vi "Axis_Offset.vi"(3 "Position In":sgl[](array[numeric])=[0.0, 0.0, 0.0] format="%#.2f", 4 "Axis":T1, 5 "Roll-Pitch-Yaw":sgl[](array[numeric]) caption="Model       Roll         Pitch        Yaw (deg)" format="%#.2f", 6 "Traverse Name":string) -> (0 "Correct array":bool, 1 "Offset":sgl, 2 "Offset Array":sgl[](array[numeric]))   [LabVIEW 2022 SP3]
uses:
  Route mapping/Axis.ctl
  Globals/Constants_global.vi
  Globals/Trav_pos_global.vi
  Globals/Meas_global.vi
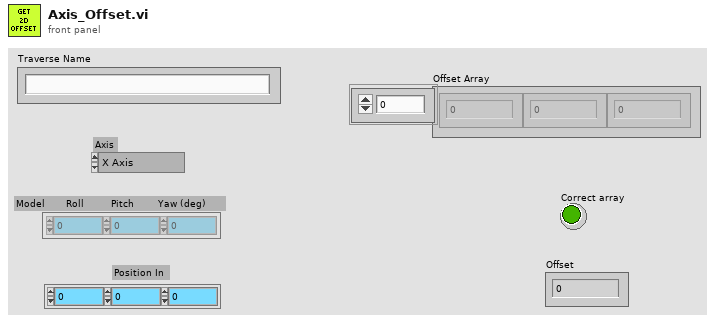
[diagram p1: front panel]
types:
  T1 = typedef "Axis.ctl" = enum16{"X Axis", "X Axis -ve", "Y Axis", "Y Axis -ve", "Z Axis", "Z Axis -ve"}
  T2 = enum16{"To Traverse Coordinates", "To User Coordinates"}
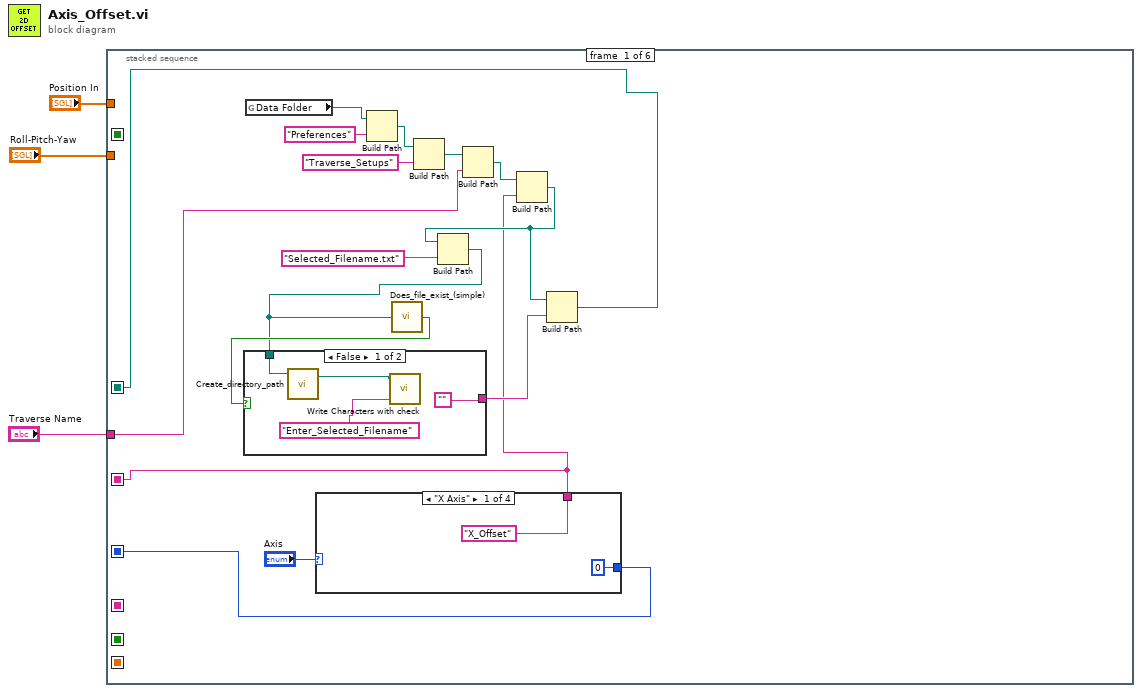
[diagram p0: block diagram]
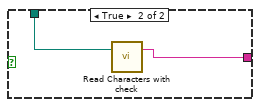
[diagram p2: hidden frame]
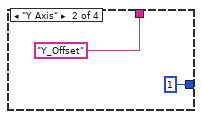
[diagram p3: hidden frame]
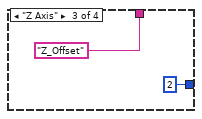
[diagram p4: hidden frame]
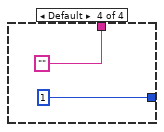
[diagram p5: hidden frame]
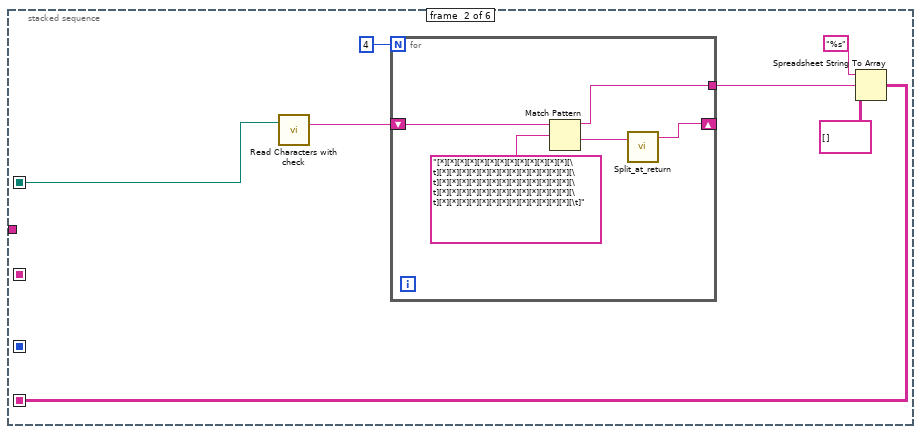
[diagram p6: hidden frame]
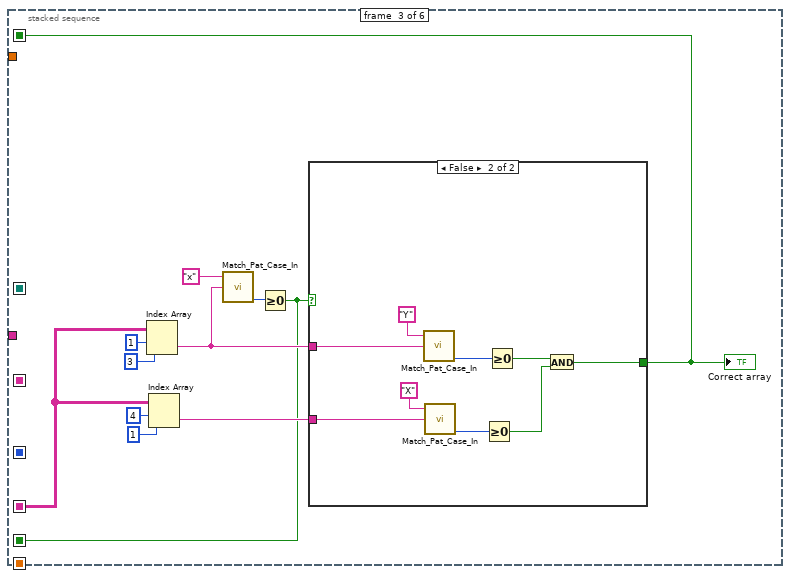
[diagram p7: hidden frame]
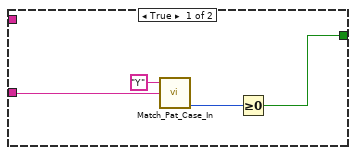
[diagram p8: hidden frame]
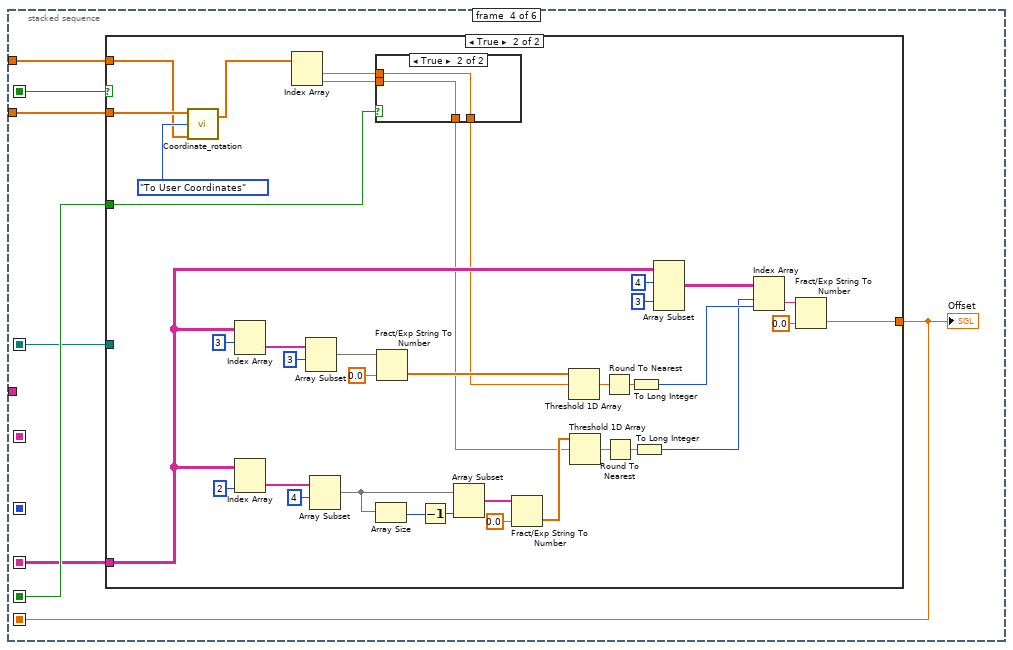
[diagram p9: hidden frame]
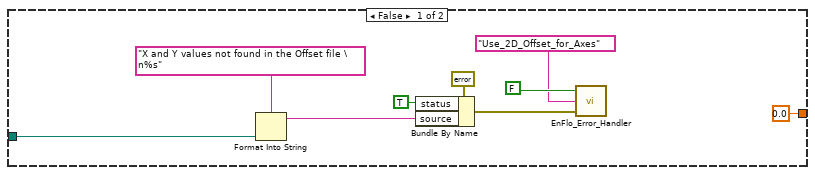
[diagram p10: hidden frame]
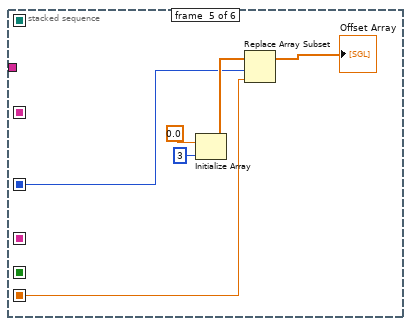
[diagram p12: hidden frame]
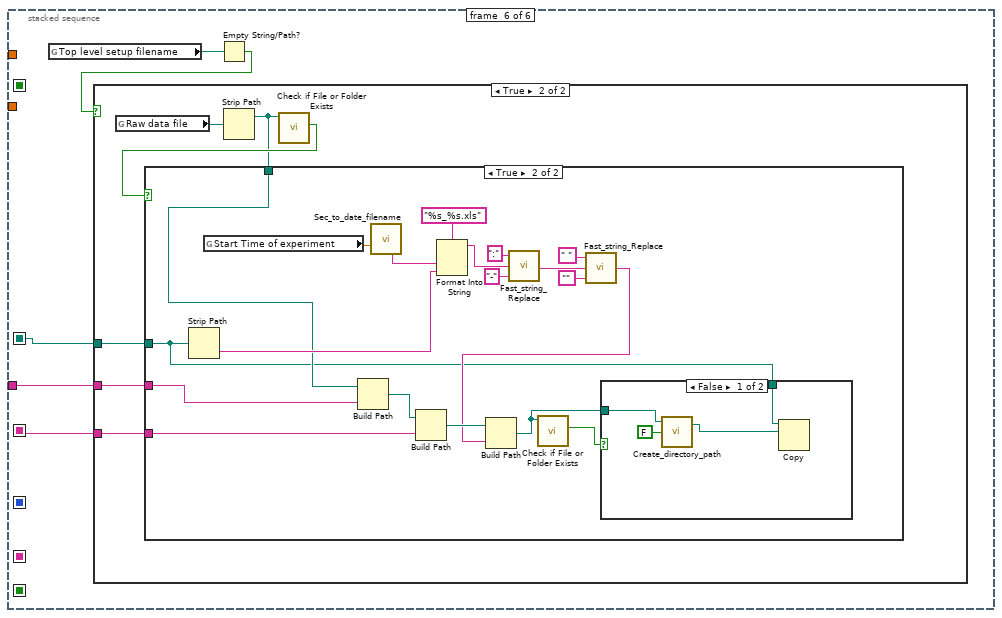
[diagram p13: hidden frame]
diagram:
  n1 = stacked-sequence {
    seq-local: [_ w36 _ _ _ _] -> [_ _ w51 w71 _ _]
    seq-local: [_ _ w47 _ _ _] -> [_ _ _ w76 _ _]
    seq-local: [_ _ _ w73 _ _] -> [_ _ _ _ w127 _]
    seq-local: [_ _ w46 _ _ _] -> [_ _ _ w74 _ _]
    seq-local: [w7 _ _ _ _ _] -> [_ w35 _ w72 _ w135]
    seq-local: [w6 _ _ _ _ _] -> [_ _ _ _ w129 _]
    seq-local: [w4 _ _ _ _ _] -> [_ _ _ _ _ w133]
    tunnel: "Position In" -> [_ _ _ w75 _ _]
    tunnel: "Roll-Pitch-Yaw" -> [_ _ _ w70 _ _]
    tunnel: "Traverse Name" -> [w5 _ _ _ _ w134]
    frame #0 {
      n2 = global read "Constants_global.vi" "Data Folder"() -> (w9:path)
      n3 = case shown="\"X Axis\"" "Axis" {
        tunnel: ["X_Offset" ("name or relative path") "Y_Offset" ("name or relative path") "Z_Offset" ("name or relative path") "" ("name or relative path")] -> w4
        tunnel: [0 ("index") 1 ("index") 2 ("index") 1 ("index")] -> w6
        frame "X Axis" {
        }
        frame "Y Axis" {
        }
        frame "Z Axis" {
        }
        frame Default {
        }
      }
      n4 = Build Path(base path=w9, name or relative path="Preferences") -> (appended path=w11:path)
      n5 = Build Path(base path=w11, name or relative path="Traverse_Setups") -> (appended path=w12:path)
      n6 = Build Path(base path=w12, name or relative path=w5) -> (appended path=w15:path)
      n7 = Build Path(base path=w15, name or relative path=w4) -> (appended path=w16:path)
      n8 = Build Path(base path=w16, name or relative path="Selected_Filename.txt" ("Substring")) -> (appended path=w17:path)
      n9 = call "Does_file_exist_(simple).vi"("Pathname"=w17) -> ("exists?"=w18:bool)
      n10 = case shown="False" w18 {
        tunnel: w17 -> [w23 w25]
        tunnel: ["" w24] -> w19
        frame False {
          n11 = call "Create_directory_path.vi"("Path name"=w23) -> ("Path name Out"=w21:path)  [unwired: 2 in, 1 out]
          n12 = call "Write Characters with check.vi"("String to Write"="Enter_Selected_Filename" ("Substring"), "file (use dialog)"=w21) -> ()  [unwired: 2 in, 1 out]
        }
        frame True {
          n13 = call "Read Characters with check.vi"("file (use dialog)"=w25) -> ("Read String"=w24:string)  [unwired: 1 in, 1 out]
        }
      }
      n14 = Build Path(base path=w16, name or relative path=w19) -> (appended path=w7:path)
    }
    frame #1 {
      n15 = call "Read Characters with check.vi"("file (use dialog)"=w35) -> ("Read String"=w34:string)  [unwired: 1 in, 1 out]
      n16 = for {
        N: 4 -> [_]
        shift-right: [w42] -> _
        shift-left: w34 -> [w43]
        tunnel: [w41] -> w38
        n17 = Match Pattern(string=w43, regular expression="[*][*][*][*][*][*][*][*][*][*][*][*][*][\t][*][*][*][*][*][*][*][*][*][*][*][*][*][\t][*][*][*][*][*][*][*][*][*][*][*][*][*][\t][*][*][*][*][*][*][*][*][*][*][*][*][*][\t][*][*][*][*][*][*][*][*][*][*][*][*][*][\t]" ("String")) -> (before substring=w41:string, after substring=w44:string)  [unwired: 3 out]
        n18 = call "Split_at_return.vi"("String"=w44) -> ("after substring"=w42:string)  [unwired: 1 in, 3 out]
      }
      n19 = Spreadsheet String To Array(format string="%s", spreadsheet string=w38, array type (2D Dbl)=string[][] []) -> (array=w36:string[][])  [unwired: 1 in]
    }
    frame #2 {
      n20 = Index Array(array=w51, index (row)=1, index (col)=3) -> (element=w49:string)
      n21 = Index Array(array=w51, index (row)=4, index (col)=1) -> (element=w50:string)
      n22 = call "Match_Pat_Case_In.vi"("String to match"="x", "String"=w49) -> ("offset past match"=w48:i32)  [unwired: 1 in, 3 out]
      n23 = Greater Or Equal To 0?(x=w48) -> (x >= 0?=w47:bool)
      n24 = case shown="False" w47 {
        tunnel: w50 -> [w59 w68]
        tunnel: w49 -> [_ w66]
        tunnel: [w57 w61] -> w46
        frame True {
          n25 = call "Match_Pat_Case_In.vi"("String to match"="Y", "String"=w59) -> ("offset past match"=w58:i32)  [unwired: 1 in, 3 out]
          n26 = Greater Or Equal To 0?(x=w58) -> (x >= 0?=w57:bool)
        }
        frame False {
          n27 = call "Match_Pat_Case_In.vi"("String to match"="Y", "String"=w66) -> ("offset past match"=w65:i32)  [unwired: 1 in, 3 out]
          n28 = call "Match_Pat_Case_In.vi"("String to match"="X", "String"=w68) -> ("offset past match"=w64:i32)  [unwired: 1 in, 3 out]
          n29 = Greater Or Equal To 0?(x=w64) -> (x >= 0?=w63:bool)
          n30 = Greater Or Equal To 0?(x=w65) -> (x >= 0?=w62:bool)
          n31 = And(x=w62, y=w63) -> (x .and. y?=w61:bool)
        }
      }
      "Correct array" <- w46
    }
    frame #3 {
      n32 = case shown="True" w74 {
        tunnel: w71 -> [_ w108]
        tunnel: w76 -> [_ w107]
        tunnel: [sgl 0.0 w102] -> w73
        tunnel: w75 -> [_ w87]
        tunnel: w72 -> [w79 _]
        tunnel: w70 -> [_ w88]
        frame False {
          n33 = Format Into String(format string="X and Y values not found in the Offset file \n%s", w79) -> (resulting string=w77:string)  [unwired: 2 in, 1 out]
          n34 = Bundle By Name(cluster=errorcluster {"status"=FALSE, "code"=0, "source"=""} ("error in (no error)"), "status"=TRUE, "source"=w77) -> (w82:errorcluster)
          n35 = call "EnFlo_Error_Handler.vi"("error in (no error)"=w82, "Error Type"="Use_2D_Offset_for_Axes", "Dialog Box (F)"=FALSE ("Dialog Box (T)")) -> ()  [unwired: 1 in, 2 out]
        }
        frame True {
          n36 = call "Coordinate_rotation.vi"("Roll-Pitch-Yaw"=w88, "Input Position"=w87, "Mode"=T2."To User Coordinates") -> ("Output Position"=w86:sgl[])  [unwired: 2 in, 1 out]
          n37 = Index Array(array=w108, index (row)=3) -> (element=w121:string[])  [unwired: 1 in]
          n38 = Index Array(array=w108, index (col)=2 ("index (row)")) -> (element=w117:string[])  [unwired: 1 in]
          n39 = Index Array(array=w86) -> (element #1=w104:sgl, element #2=w103:sgl)  [unwired: 2 in]
          n40 = Array Subset(array=w121, index=3) -> (w114:string[])  [unwired: 1 in]
          n41 = Array Subset(array=w117, index=4) -> (w94:string[])  [unwired: 1 in]
          n42 = case shown="True" w107 {
            tunnel: w104 -> [w124 w126]
            tunnel: [w123 w126] -> w106
            tunnel: [w124 w125] -> w105
            tunnel: w103 -> [w123 w125]
            frame False {
            }
            frame True {
            }
          }
          n43 = Array Size(array=w94) -> (size(s)=w96:i32)
          n44 = Fract/Exp String To Number(string=w114, default (0 dbl)=sgl 0.0 ("default (0 DBL)")) -> (number=w113:sgl[])  [unwired: 2 in, 1 out]
          n45 = Decrement(x=w96) -> (x-1=w95:i32)
          n46 = Array Subset(array=w94, length=w95) -> (w93:string[])  [unwired: 1 in]
          n47 = Fract/Exp String To Number(string=w93, default (0 dbl)=sgl 0.0 ("default (0 DBL)")) -> (number=w110:sgl[])  [unwired: 2 in, 1 out]
          n48 = Threshold 1D Array(2:w106, 3:w113) -> (0:w112:sgl)  [unwired: 1 in]
          n49 = Threshold 1D Array(2:w105, 3:w110) -> (0:w111:sgl)  [unwired: 1 in]
          n50 = Round To Nearest(number=w112) -> (nearest integer value=w101:sgl)
          n51 = Round To Nearest(number=w111) -> (nearest integer value=w100:sgl)
          n52 = To Long Integer(number=w101) -> (32bit integer=w98:i32)
          n53 = To Long Integer(number=w100) -> (32bit integer=w97:i32)
          n54 = Array Subset(array=w108, index (row)=4 ("index"), index (col)=3 ("index")) -> (w99:string[][])  [unwired: 2 in]
          n55 = Index Array(array=w99, index (row)=w97, index (col)=w98) -> (element=w109:string)
          n56 = Fract/Exp String To Number(string=w109, default (0 dbl)=sgl 0.0 ("default (0 DBL)")) -> (number=w102:sgl)  [unwired: 2 in, 1 out]
        }
      }
      "Offset" <- w73
    }
    frame #4 {
      n57 = Initialize Array(sgl 0.0, 3 ("dimension size")) -> (w130:sgl[])
      n58 = Replace Array Subset(array=w130, new element=w127, index=w129) -> (→"Offset Array":sgl[])
    }
    frame #5 {
      n59 = global read "Trav_pos_global.vi" "Top level setup filename"() -> (w137:path)
      n60 = Empty String/Path?(string/path=w137) -> (empty?=w136:bool)
      n61 = case shown="True" w136 {
        tunnel: w135 -> [_ w141]
        tunnel: w134 -> [_ w139]
        tunnel: w133 -> [_ w138]
        frame False {
        }
        frame True {
          n62 = global read "Meas_global.vi" "Raw data file"() -> (w143:path)
          n63 = Strip Path(path=w143) -> (stripped path=w140:path)  [unwired: 1 out]
          n64 = call <vilib>:"Check if File or Folder Exists.vi"("path"=w140) -> ("file or folder exists?"=w142:bool)  [unwired: 8 in, 2 out]
          n65 = case shown="True" w142 {
            tunnel: w141 -> [_ w145]
            tunnel: w140 -> [_ w153]
            tunnel: w139 -> [_ w152]
            tunnel: w138 -> [_ w150]
            frame False {
            }
            frame True {
              n66 = Strip Path(path=w145) -> (name=w154:string)  [unwired: 1 out]
              n67 = global read "Meas_global.vi" "Start Time of experiment"() -> (w155:dbl)
              n68 = Build Path(base path=w153, name or relative path=w152) -> (appended path=w151:path)
              n69 = call "Sec_to_date_filename.vi"("ss1904"=w155) -> ("YYYY-mm-DD HH:MM"=w144:string)  [unwired: 5 in, 9 out]
              n70 = Build Path(base path=w151, name or relative path=w150) -> (appended path=w149:path)
              n71 = Format Into String(format string="%s_%s.xls", w144, w154) -> (resulting string=w160:string)  [unwired: 2 in, 1 out]
              n72 = call "Fast_string_Replace.vi"("Replace match with:"="-", "Input String"=w160, "matchThis"=":" ("regular expression")) -> ("Output String"=w157:string)  [unwired: 1 in, 1 out]
              n73 = call "Fast_string_Replace.vi"("Replace match with:"="", "Input String"=w157, "matchThis"=" " ("regular expression")) -> ("Output String"=w148:string)  [unwired: 1 in, 1 out]
              n74 = Build Path(base path=w149, name or relative path=w148) -> (appended path=w146:path)
              n75 = call <vilib>:"Check if File or Folder Exists.vi"("path"=w146) -> ("file or folder exists?"=w147:bool)  [unwired: 8 in, 2 out]
              n76 = case shown="False" w147 {
                tunnel: w146 -> [w165 _]
                tunnel: w145 -> [w164 _]
                frame False {
                  n77 = call "Create_directory_path.vi"("Dialog Box"=FALSE, "Path name"=w165) -> ("Path name Out"=w163:path)  [unwired: 1 in, 1 out]
                  n78 = Copy(10:w163, 11:w164) -> ()  [unwired: 3 in, 3 out]
                }
                frame True {
                }
              }
            }
          }
        }
      }
    }
  }
